vi "Create.vi"(8 "error in (no error)":errorcluster) -> (0 "error out":errorcluster, 3 "Result out":refnum<class "Result.lvclass">)   [LabVIEW 2017, in "Futures.lvlib" / "Result.lvclass"]
uses:
  Result.lvclass
  Result Data.ctl
  Result Type.ctl
  Result.lvclass/Result.ctl
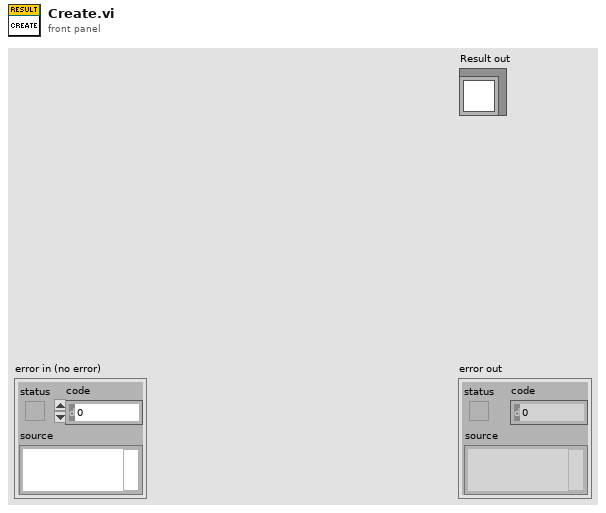
[diagram p1: front panel]
types:
  T1 = typedef "Futures.lvlib/Result.lvclass/Result Data.ctl" = cluster{"Type":T2, "Value":variant}
  T2 = typedef "Futures.lvlib/Result.lvclass/Result Type.ctl" = enum16{"Unresolved", "Ok", "Error"}
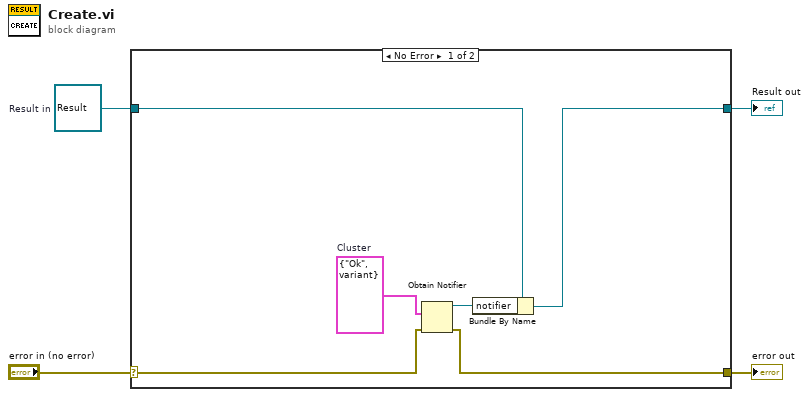
[diagram p0: block diagram]
diagram:
  w2 = refnum<class "Result.lvclass"> refnum  # Result in
  n1 = case shown="No Error" "error in (no error)" {
    selector: "error in (no error)" -> [w8 w12]
    tunnel: [w7 w12] -> w3
    tunnel: [w6 w11] -> w1
    tunnel: w2 -> [w10 w11]
    frame No Error {
      w9 = T1 {"Type"=enum."Ok", "Value"=variant}  # Cluster
      n2 = Obtain Notifier(notification data type=w9, error in (no error)=w8) -> (notifier out=w5:refnum<notifier>, error out=w7:errorcluster)  [unwired: 2 in, 1 out]
      n3 = Bundle By Name(cluster=w10, "notifier"=w5) -> (w6:refnum<class "Result.lvclass">)
    }
    frame Error {
    }
  }
  "error out" <- w3
  "Result out" <- w1
